vi "SVPO FFT Spectrum (Complex).vi"   [LabVIEW 2017]
doc: "Computes the Fast Fourier Transform (FFT) spectrum of <B>scaled signal [EU]</B>. This VI returns FFT results as the complex form of the FFT spectrum. Wire data to the <B>scaled signal [EU]</B> input to determine the polymorphic instance to use or manually select the instance.\n\nThis VI is designed to operate on a single block of data, as opposed to being called repeatedly to operate on a continuous flow of data. Use this VI after performing a finite acquisition, or when you need to analyze a single block of data without previously analyzed blocks affecting the result."
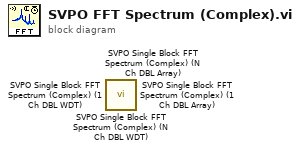
[diagram p0: block diagram]
diagram:
  n1 = call <vilib>:"SVPO Single Block FFT Spectrum (Complex) (N Ch DBL WDT).vi"() -> ()  [unwired: 19 in, 1 out]
  n2 = call <vilib>:"SVPO Single Block FFT Spectrum (Complex) (N Ch DBL Array).vi"() -> ()  [unwired: 19 in, 1 out]
  n3 = call <vilib>:"SVPO Single Block FFT Spectrum (Complex) (1 Ch DBL WDT).vi"() -> ()  [unwired: 19 in, 1 out]
  n4 = call <vilib>:"SVPO Single Block FFT Spectrum (Complex) (1 Ch DBL Array).vi"() -> ()  [unwired: 19 in, 1 out]
